vi "DOG.vi"(1 "pixel cached Memory":refnum<k21>, 4 "Data in":u8, 5 "DV in":bool, 6 "Height":u16, 8 "Width":u16, 9 "DelayRowCount":i8, 10 "Rows":u16, 12 "Cols":u16) -> (11 "out Row":u16, 14 "GaussianFilterData out":u8, 17 "DV out":bool)   [LabVIEW 2016]
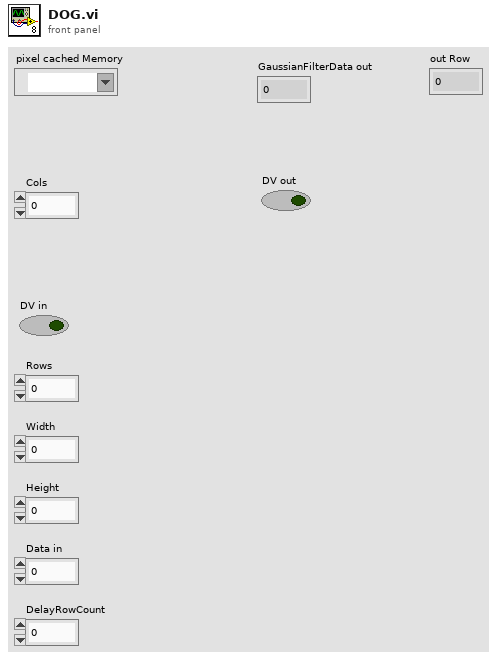
[diagram p1: front panel]
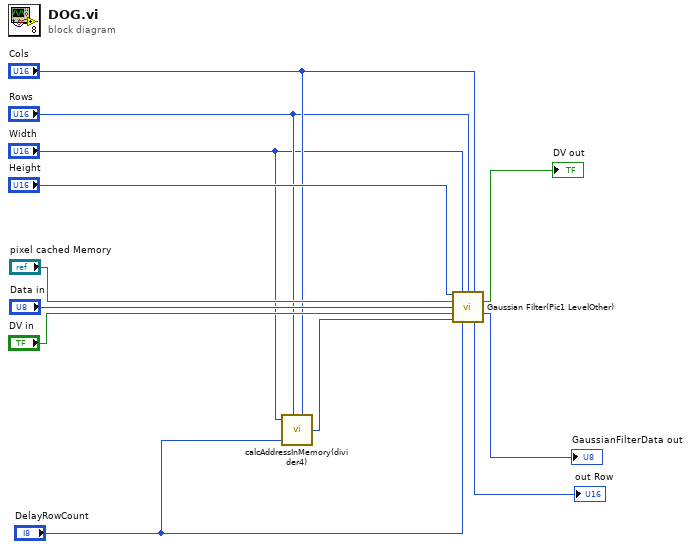
[diagram p0: block diagram]
diagram:
  n1 = call "calcAddressInMemory(divider4).vi"("Width"="Width", "Rows"="Rows", "delayRowCount"="DelayRowCount", "Cols"="Cols") -> ("addressInMemory"=w5:u16)  [unwired: 5 in]
  n2 = call "Gaussian Filter(Pic1 LevelOther).vi"("Height"="Height", "Width"="Width", "Rows"="Rows", "Cols"="Cols", "Memory in"="pixel cached Memory", "Data in"="Data in", "DV in"="DV in", "Address In"=w5, "DelayRowCount"="DelayRowCount") -> ("DV out"=→"DV out":bool, "Data Out"=→"GaussianFilterData out":u8, "out Row"=→"out Row":u16)  [unwired: 4 in]
